vi "写号工具.vi"() -> ()   [LabVIEW 2018]
doc: "欢迎使用飞图同辉对讲机账号写入工具，对于新芯片fly380s-8910。"
uses:
  <vilib>/Utility/error.llb/DialogType.ctl
  <vilib>/Instr/_visa.llb/VISA Configure Serial Port (Instr).vi
  <vilib>/Instr/_visa.llb/VISA Find Search Mode.ctl
panel:
  in  "端口号":refnum<visa-resource-name>
  out "串口状态":bool
  out "串口COM":refnum<visa-resource-name>
  in  "端口号":u16(ring) items=["COM1", "COM2", "COM5", "COM6", "COM8", "COM9", "COM10", "COM11", "COM12", "COM13", "COM14", "COM15", "COM16", "COM17", "COM18", "COM19", "COM20", "COM21"]
  out "错误状态":bool=TRUE
  out "状态":string
  in  "密码":string(combo)
  in  "账号":string(combo)
  in  "端口号":string(combo)
  in  "ip地址":string(combo)
  out "run":bool
  out "stop":bool
  in  "打开串口":bool
  in  "清空显示":bool
  in  "波特率":u16(ring) items=["115200"=65535, "57600"=57600, "56000"=56000, "38400"=38400, "19200"=19200, "14400"=14400, "9600"=9600, "4800"=4800, "2400"=2400]
  in  "数据位":u16(ring) items=["8"=8, "7"=7, "6"=6, "5"=5]
  in  "发送":bool
  in  "显示区":string
  # "飞图同辉写号工具"
  # "①账号及密码请您向飞图相关人员申请；\n②账号及密码只列出首尾项，中间项均可用；\n③感谢您的使用。"
  # "①ip及端口号请您不要擅自修改；\n②请与飞图相关人员沟通确认；\n③感谢您的使用。"
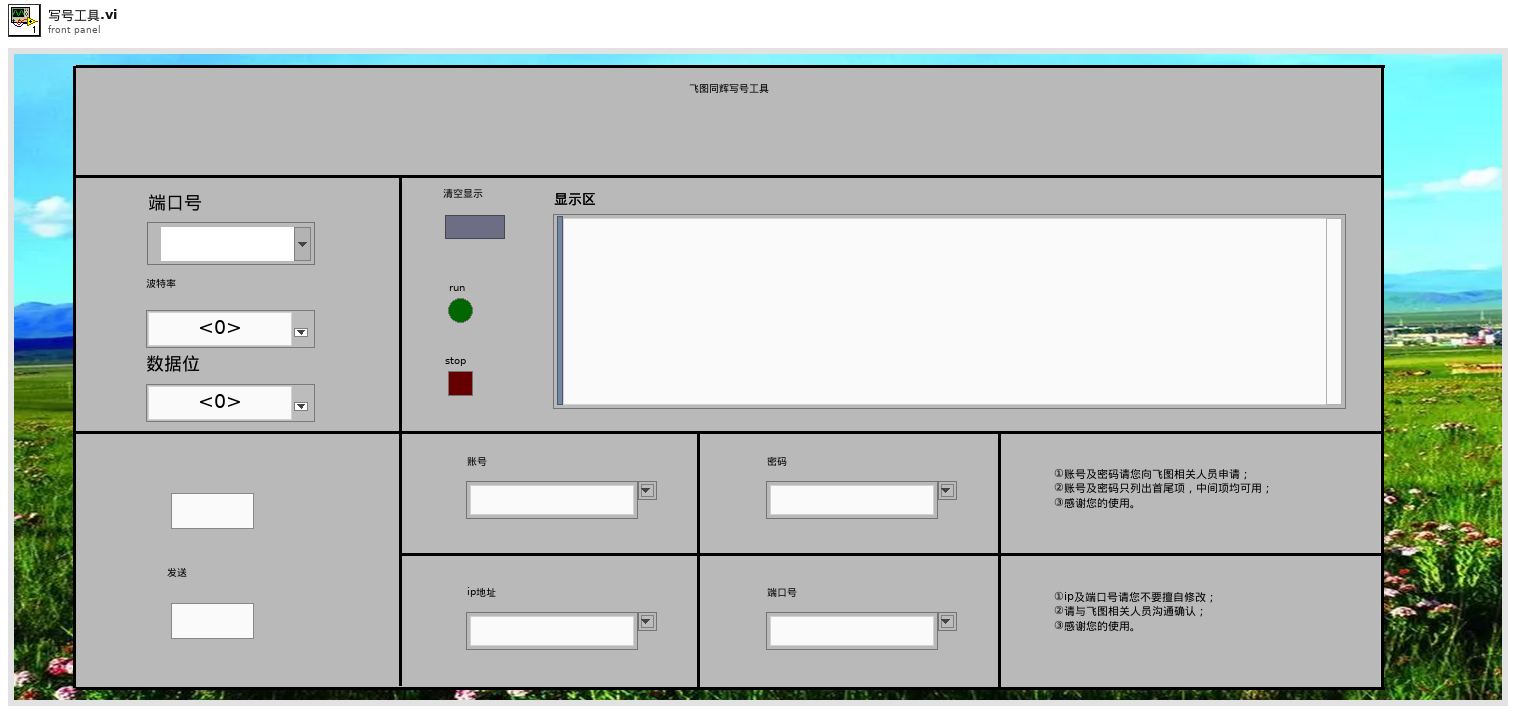
[diagram p1: front panel]
types:
  T1 = typedef "VISA Find Search Mode.ctl" = u32
  T2 = typedef "DialogType.ctl" = u16
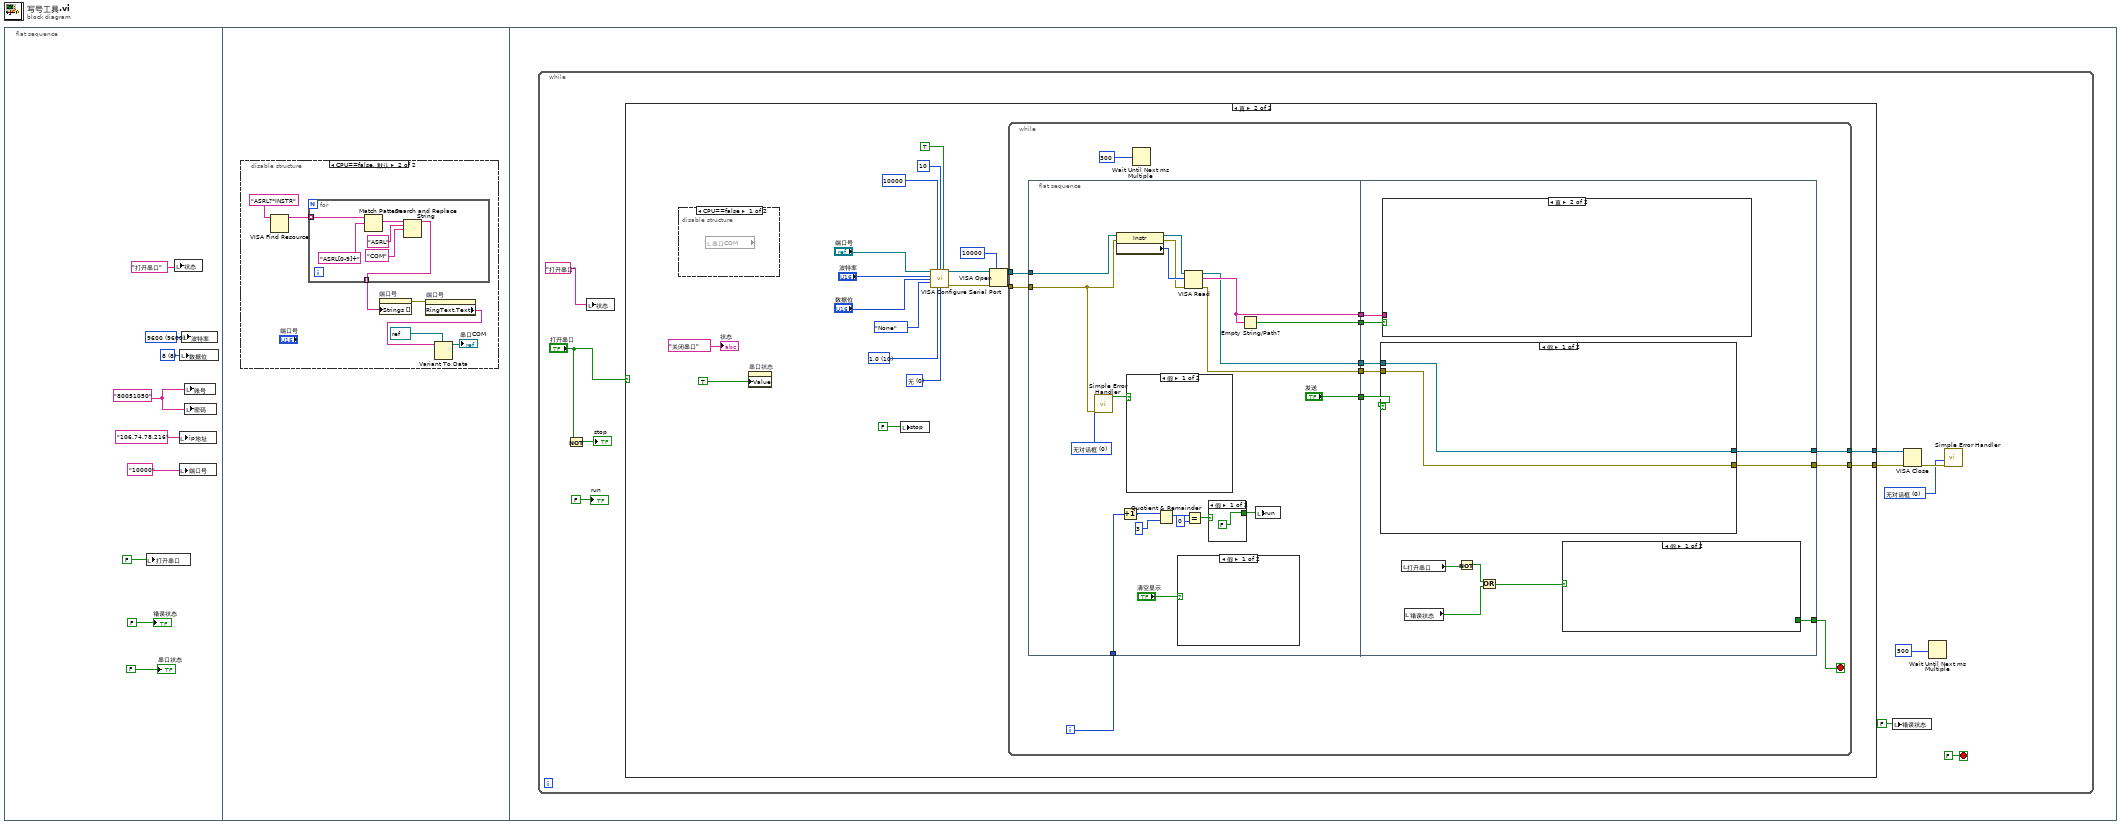
[diagram p0: block diagram]
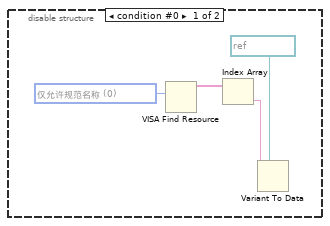
[diagram p2: hidden frame]
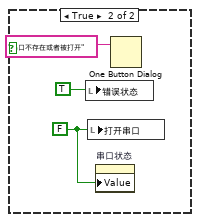
[diagram p5: hidden frame]
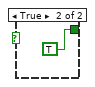
[diagram p6: hidden frame]
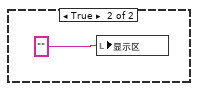
[diagram p7: hidden frame]
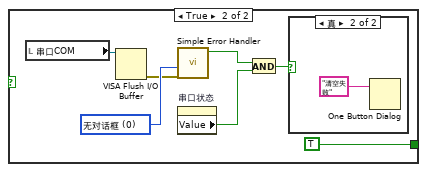
[diagram p8: hidden frame]
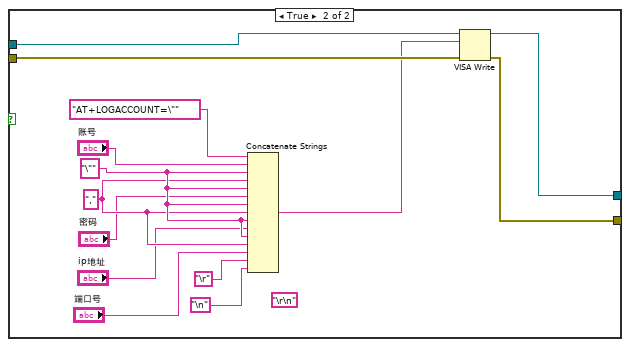
[diagram p10: hidden frame]
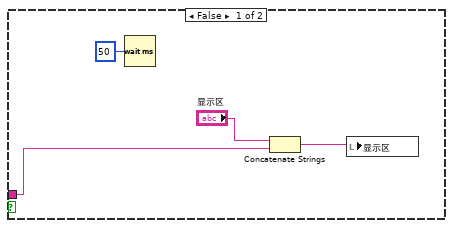
[diagram p11: hidden frame]
diagram:
  n1 = flat-sequence {
    frame #0 {
      w4 = u16 8 items=["8"=8, "7"=7, "6"=6, "5"=5] ("数据位")
      w5 = u16 9600 items=["115200"=65535, "57600"=57600, "56000"=56000, "38400"=38400, "19200"=19200, "14400"=14400, "9600"=9600, "4800"=4800, "2400"=2400] ("波特率")
      w6 = "80051050"
      n2 = local write "打开串口"(FALSE) -> ()
      n3 = local write "状态"("打开串口") -> ()
      n4 = local write "ip地址"("106.74.78.216") -> ()
      n5 = local write "端口号"("10000") -> ()
      n6 = local write "数据位"(w4) -> ()
      n7 = local write "波特率"(w5) -> ()
      n8 = local write "账号"(w6) -> ()
      n9 = local write "密码"(w6) -> ()
      "错误状态" <- FALSE
      "串口状态" <- FALSE
    }
    frame #1 {
      n10 = disable-structure shown="CPU==false, 默认" {
        frame condition #0 {
          w14 = T1 0 items=["仅允许规范名称"=0, "只允许别名"=2, "包含匹配别名"=3, "包含所有别名"=4] ("Search Mode")
          n11 = VISA Find Resource(10:w14) -> (3:w13:string[])  [unwired: 2 in, 2 out]
          n12 = Index Array(array=w13) -> (element=w12:string)  [unwired: 1 in]
          n13 = Variant To Data(type=refnum<visa-resource-name> "COM1" ("VISA资源名称"), Variant=w12) -> (data=w11:refnum<visa-resource-name>)  [unwired: 1 in, 1 out]
        }
        frame condition #1 (active) {
          n14 = VISA Find Resource(11:"ASRL?*INSTR" ("表达式(\"?*\")")) -> (3:w20:string[])  [unwired: 2 in, 2 out]
          n15 = for {
            tunnel: w20 -> [w27] mode=indexing
            tunnel: [w23] -> w19 mode=indexing
            n16 = Match Pattern(string=w27, regular expression="ASRL[0-9]+" ("正则表达式")) -> (match substring=w22:string)  [unwired: 1 in, 3 out]
            n17 = Search and Replace String(input string=w22, search string="ASRL" ("搜索字符串"), replace string="COM" ("替换字符串(\"\")")) -> (result string=w23:string)  [unwired: 5 in, 3 out]
          }
          n18 = property on="端口号" class="Ring (严格)"("Strings []"=w19) -> (error out=w18:errorcluster)  [unwired: 2 in, 1 out]
          n19 = property on="端口号" class="Ring (严格)"(error in=w18) -> ("RingText.Text"=w17:string)  [unwired: 1 in, 2 out]
          n20 = Variant To Data(type=refnum<visa-resource-name> refnum ("VISA resource name"), Variant=w17) -> (data=→"串口COM":refnum<visa-resource-name>)  [unwired: 1 in, 1 out]
        }
      }
    }
    frame #2 {
      n21 = while {
        stop <- FALSE stop-if-true
        w28 = T2 0 items=["无对话框", "确定信息", "继续或停止信息", "确定信息＋警告", "继续/停止+警告"] ("type of dialog (OK msg:1)")
        n22 = Not(x="打开串口") -> (.not. x?=→"stop":bool)
        n23 = local write "状态"("打开串口") -> ()
        n24 = case shown="真" "打开串口" {
          tunnel: [_ w42] -> w30
          tunnel: [_ w41] -> w31
          frame False {
          }
          frame True {
            w50 = u16 10 items=["1.0"=10, "1.5"=15, "2.0"=20] ("stop bits (10: 1 bit)")
            w51 = u16 0 items=["无", "XON/XOFF", "RTS/CTS", "XON/XOFF & RTS/CTS", "DTR/DSR", "XON/XOFF & DTR/DSR"] ("flow control (0:none)")
            n25 = disable-structure shown="CPU==false" {
              frame condition #0 {
                n26 = local read "串口COM"() -> ()  [unwired: 1 out]
              }
              frame condition #1 (active) {
              }
            }
            n27 = property on="串口状态" class="Bool (严格)"("Value"=TRUE) -> ()  [unwired: 2 in, 2 out]
            n28 = local write "stop"(FALSE) -> ()
            n29 = call-poly "VISA Configure Serial Port"("VISA resource name"="端口号", "timeout (10sec)"=u32 10000, "termination char\n(0xA = '\\n' = LF)"=u8 10 ("termination char\n(0xA = '\\n' = LF)"), "Enable Termination\nChar (T)"=TRUE ("Enable Termination\nChar (T)"), "baud rate (9600)"="波特率", "data bits (8)"="数据位", "parity (0:none)"=enum16{"None", "Odd", "Even", "Mark", "Space"}."None", "stop bits (10: 1 bit)"=w50, "flow control (0:none)"=w51) -> ("VISA resource name out"=w55:refnum<visa-resource-name>, "error out"=w54:errorcluster)  [unwired: 5 in]
            n30 = VISA Open(timeout (0)=u32 10000 ("VISA打开超时（0）"), error in (no error)=w54, VISA resource name=w55) -> (VISA resource name=w57:refnum<visa-resource-name>, error out=w56:errorcluster)  [unwired: 2 in]
            n31 = while {
              tunnel: w57 -> [w68]
              tunnel: w56 -> [w66]
              tunnel: [w60] -> w42
              tunnel: [w59] -> w41
              i -> [w67]
              stop <- w58 stop-if-true
              n32 = flat-sequence {
                tunnel: w68 -> [w85]
                tunnel: w67 -> [w81]
                tunnel: w66 -> [w71]
                tunnel: [w88] -> w65
                tunnel: [w87] -> w64
                tunnel: ["发送"] -> w63
                tunnel: [w84] -> w62
                tunnel: [w82] -> w61
                tunnel: w65 -> [w105]
                tunnel: w64 -> [w104]
                tunnel: w63 -> [w106]
                tunnel: w62 -> [w102]
                tunnel: w61 -> [w103]
                tunnel: [w101] -> w60
                tunnel: [w100] -> w59
                tunnel: [w99] -> w58
                frame #0 {
                  w70 = T2 0 items=["无对话框", "确定信息", "继续或停止信息", "确定信息＋警告", "继续/停止+警告"] ("type of dialog (OK msg:1)")
                  n33 = call <vilib>:"Simple Error Handler.vi"("type of dialog (OK msg:1)"=w70, "error in (no error)"=w71) -> ("error?"=w74:bool)  [unwired: 3 in, 4 out]
                  n34 = property class="Instr"(reference=w85, error in=w71) -> (reference out=w73:refnum<visa-resource-name>, error out=w72:errorcluster, "Serial Settings:Number of Bytes at Serial Port"=w89:u32)
                  n35 = Increment(x=w81) -> (x+1=w80:i32)
                  n36 = case shown="假" w74 {
                    frame False {
                    }
                    frame True {
                      w90 = FALSE
                      n37 = local write "错误状态"(TRUE) -> ()
                      n38 = local write "打开串口"(w90) -> ()
                      n39 = property on="串口状态" class="Bool (严格)"("Value"=w90) -> ()  [unwired: 2 in, 2 out]
                      n40 = One Button Dialog(message="串口不存在或者被打开" ("消息")) -> ()  [unwired: 1 in, 1 out]
                    }
                  }
                  n41 = Quotient & Remainder(x=w80, y=3) -> (x-y*floor(x/y)=w78:i32)  [unwired: 1 out]
                  n42 = case shown="假" "清空显示" {
                    frame False {
                    }
                    frame True {
                      n43 = local write "显示区"("") -> ()
                    }
                  }
                  n44 = VISA Read(VISA resource name=w73, byte count=w89, error in (no error)=w72) -> (VISA resource name out=w82:refnum<visa-resource-name>, read buffer=w87:string, error out=w84:errorcluster)  [unwired: 1 out]
                  n45 = Equal?(x=w78, y=0) -> (x = y?=w76:bool)
                  n46 = case shown="假" w76 {
                    tunnel: [FALSE TRUE] -> w75
                    frame False {
                    }
                    frame True {
                    }
                  }
                  n47 = Empty String/Path?(string/path=w87) -> (empty?=w88:bool)
                  n48 = local write "run"(w75) -> ()
                }
                frame #1 {
                  n49 = case shown="假" w106 {
                    tunnel: w103 -> [w117 w131]
                    tunnel: w102 -> [w116 w130]
                    tunnel: [w117 w129] -> w101
                    tunnel: [w116 w128] -> w100
                    frame False {
                    }
                    frame True {
                      (unwired) "\r\n"
                      w125 = ","
                      w126 = "\""
                      n50 = Concatenate Strings("AT+LOGACCOUNT=\"", "账号", w126, w125, w126, "密码", w126, w125, w126, "ip地址", w126, w125, "端口号", "\r", "\n") -> (w118:string)
                      n51 = VISA Write(VISA resource name=w131, write buffer=w118, error in (no error)=w130) -> (VISA resource name out=w129:refnum<visa-resource-name>, error out=w128:errorcluster)  [unwired: 1 out]
                    }
                  }
                  n52 = case shown="真" w105 {
                    tunnel: w104 -> [w134 _]
                    frame False {
                      n53 = Wait (ms)(milliseconds to wait=u32 50 ("等待时间（毫秒）")) -> ()  [unwired: 1 out]
                      n54 = Concatenate Strings("显示区", w134) -> (w132:string)
                      n55 = local write "显示区"(w132) -> ()
                    }
                    frame True {
                    }
                  }
                  n56 = local read "打开串口"() -> (w107:bool)
                  n57 = local read "错误状态"() -> (w97:bool)
                  n58 = Not(x=w107) -> (.not. x?=w98:bool)
                  n59 = Or(x=w98, y=w97) -> (x .or. y?=w96:bool)
                  n60 = case shown="假" w96 {
                    tunnel: [_ TRUE] -> w99
                    frame False {
                    }
                    frame True {
                      w113 = T2 0 items=["无对话框", "确定信息", "继续或停止信息", "确定信息＋警告", "继续/停止+警告"] ("type of dialog (OK msg:1)")
                      n61 = local read "串口COM"() -> (w112:refnum<visa-resource-name>)
                      n62 = VISA Flush I/O Buffer(VISA resource name=w112) -> (error out=w111:errorcluster)  [unwired: 2 in, 1 out]
                      n63 = call <vilib>:"Simple Error Handler.vi"("type of dialog (OK msg:1)"=w113, "error in (no error)"=w111) -> ("error?"=w109:bool)  [unwired: 3 in, 4 out]
                      n64 = property on="串口状态" class="Bool (严格)"() -> ("Value"=w108:bool)  [unwired: 2 in, 2 out]
                      n65 = And(x=w109, y=w108) -> (x .and. y?=w110:bool)
                      n66 = case shown="真" w110 {
                        frame False {
                        }
                        frame True {
                          n67 = One Button Dialog(message="清空失败" ("消息")) -> ()  [unwired: 1 in, 1 out]
                        }
                      }
                    }
                  }
                }
              }
              n68 = Wait Until Next ms Multiple(millisecond multiple=u32 300 ("毫秒倍数")) -> ()  [unwired: 1 out]
            }
            "状态" <- "关闭串口"
          }
        }
        n69 = local write "错误状态"(FALSE) -> ()
        n70 = VISA Close(VISA resource name=w30, error in (no error)=w31) -> (error out=w29:errorcluster)
        n71 = Wait Until Next ms Multiple(millisecond multiple=u32 500 ("毫秒倍数")) -> ()  [unwired: 1 out]
        n72 = call <vilib>:"Simple Error Handler.vi"("type of dialog (OK msg:1)"=w28, "error in (no error)"=w29) -> ()  [unwired: 3 in, 5 out]
        "run" <- FALSE
      }
    }
  }
